vi "Pre Launch Init.vi"(11 "Nested in":refnum<class "Sub Panel Actor.lvclass">) -> (0 "error out":errorcluster, 3 "Nested out":refnum<class "Sub Panel Actor.lvclass">)   [LabVIEW 2020, in "Sub Panel Actor.lvlib" / "Sub Panel Actor.lvclass"]
doc: "(<B>Filename</B>: Actor Framework.lvlib:Actor.lvclass:Pre Launch Init.vi)\n\nDefines behavior that occurs after the Launch Nested Actor method is invoked but before the actor's Actor Core method begins running.\n\nBy default, this method does nothing. A descendant class may override it to define behavior."
uses:
  Sub Panel Actor.lvclass
  Sub Panel Actor.lvclass/Sub Panel Actor.ctl
  <vilib>/ActorFramework/Actor/Actor.lvclass
  Sub Panel Actor Messages/Initialize Msg/Initialize Msg.lvclass
  C:/Program Files (x86)/National Instruments/LabVIEW 2020/vi.lib/ActorFramework/Actor/Actor.lvclass
  C:/Users/eddiews/Documents/Git Hub Repositorios/VendingMachine_ActorFramework/Sub Panel Actor.lvclass
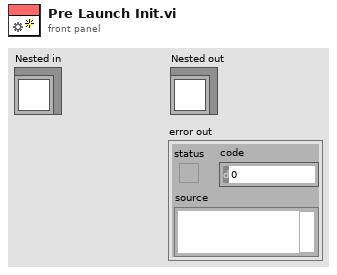
[diagram p1: front panel]
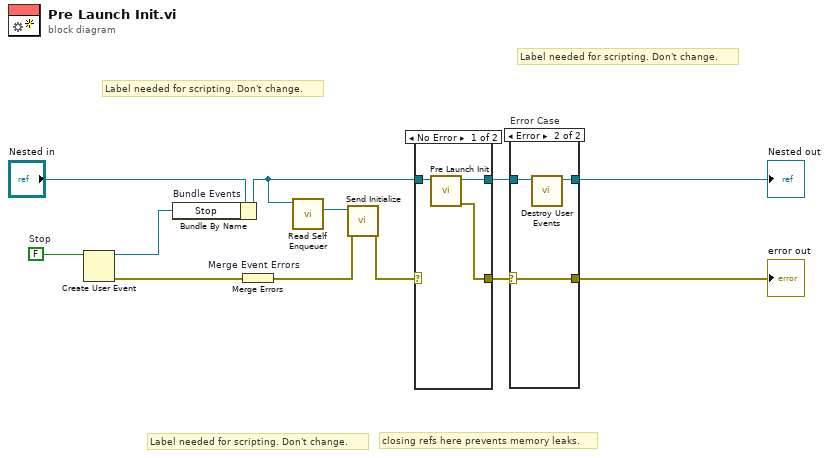
[diagram p0: block diagram]
diagram:
  w11 = FALSE  # Stop
  # "Label needed for scripting. Don't change."
  # "Label needed for scripting. Don't change."
  # "Label needed for scripting. Don't change."
  # "closing refs here prevents memory leaks."
  n1 = Create User Event(user event datatype=w11) -> (user event=w8:refnum<user-event>, error out=w10:errorcluster)  [unwired: 1 in]
  n2 = Bundle By Name "Bundle Events"(cluster="Nested in", "Stop"=w8) -> (w1:refnum<class "Sub Panel Actor.lvclass">)
  n3 = Merge Errors "Merge Event Errors"(w10) -> (w3:errorcluster)
  n4 = call <vilib>:"Read Self Enqueuer.vi"("Actor"=w1) -> ("Self Enqueuer"=w2:refnum<class "Message Enqueuer.lvclass">)  [unwired: 10 in]
  n5 = call "Send Initialize.vi"("error in (no error)"=w3, "Message Enqueuer"=w2) -> ("error out"=w4:errorcluster)  [unwired: 8 in, 1 out]
  n6 = case shown="No Error" w4 {
    selector: w4 -> [_ w17]
    tunnel: [w15 w16] -> w6
    tunnel: w1 -> [w14 w16]
    tunnel: [w13 w17] -> w5
    frame No Error {
      n7 = call-parent "Pre Launch Init.vi"("Actor in"=w14) -> ("error out"=w13:errorcluster, "Actor out"=w15:refnum<class "Sub Panel Actor.lvclass">)  [unwired: 9 in]
    }
    frame Error {
    }
  }
  n8 = case "Error Case" shown="Error" w5 {
    selector: w5 -> [w18 w22]
    tunnel: w6 -> [w19 w21]
    tunnel: [w19 w20] -> w9
    tunnel: [w18 w22] -> w7
    frame No Error {
    }
    frame Error {
      n9 = call "Destroy User Events.vi"("UI Template in"=w21) -> ("UI Template out"=w20:refnum<class "Sub Panel Actor.lvclass">)  [unwired: 10 in]
    }
  }
  "error out" <- w7
  "Nested out" <- w9
